vi "Gyro Correction.vi"(10 "Setpoint":dbl, 11 "Angle Setpoint":dbl format="%.2f") -> (2 "Correction":dbl format="%.2f", 3 "Corrected Setpoint":dbl)   [LabVIEW 2019]
uses:
  Drive Published Globals.vi
  <vilib>/addons/control/pid/pid.llb/PID (DBL).vi
  <vilib>/addons/control/pid/NI_PID_pid.lvlib
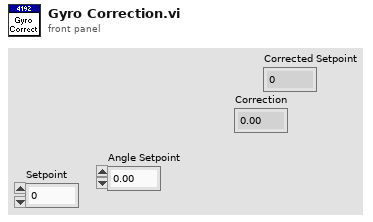
[diagram p1: front panel]
types:
  T1 = cluster{"proportional gain (Kc)":dbl, "integral time (Ti, min)":dbl, "derivative time (Td, min)":dbl}
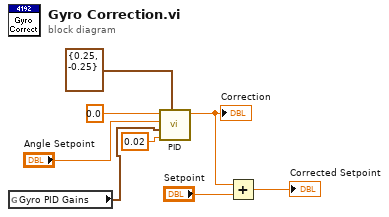
[diagram p0: block diagram]
diagram:
  n1 = global read "Drive Published Globals.vi" "Gyro PID Gains"() -> (w1:T1)
  n2 = call-poly <vilib>:"PID.vi"("output range"=cluster{"output high":dbl, "output low":dbl} {"output high"=0.25, "output low"=-0.25}, "dt (s)"=0.02, "PID gains"=w1, "process variable"="Angle Setpoint", "setpoint"=0.0 ("process variable")) -> ("output"=w6:dbl)  [unwired: 5 in, 1 out]
  "Correction" <- w6
  n3 = Add(x=w6, y="Setpoint") -> (x+y=→"Corrected Setpoint":dbl)
